vi "ReOrigin.vi"() -> ()   [LabVIEW 2018]
uses:
  <vilib>/Utility/miscctls.llb/LVPointTypeDef.ctl
  <vilib>/Utility/error.llb/DialogType.ctl
panel:
  in  "控件排布前面板.位置_前.位置":T1 caption="假设原点"
  in  "设定":bool
  out "Error Report":string
  out "Current State":string
  in  "Data Structure":T2
  in  "OK":bool
  in  "Exit Program":bool
  in  "Error":bool
  in  "Parameter":T3={"Q-HighLevel"="Q-HighLevel", "Q-Local"="Enginex", "Data"=variant}
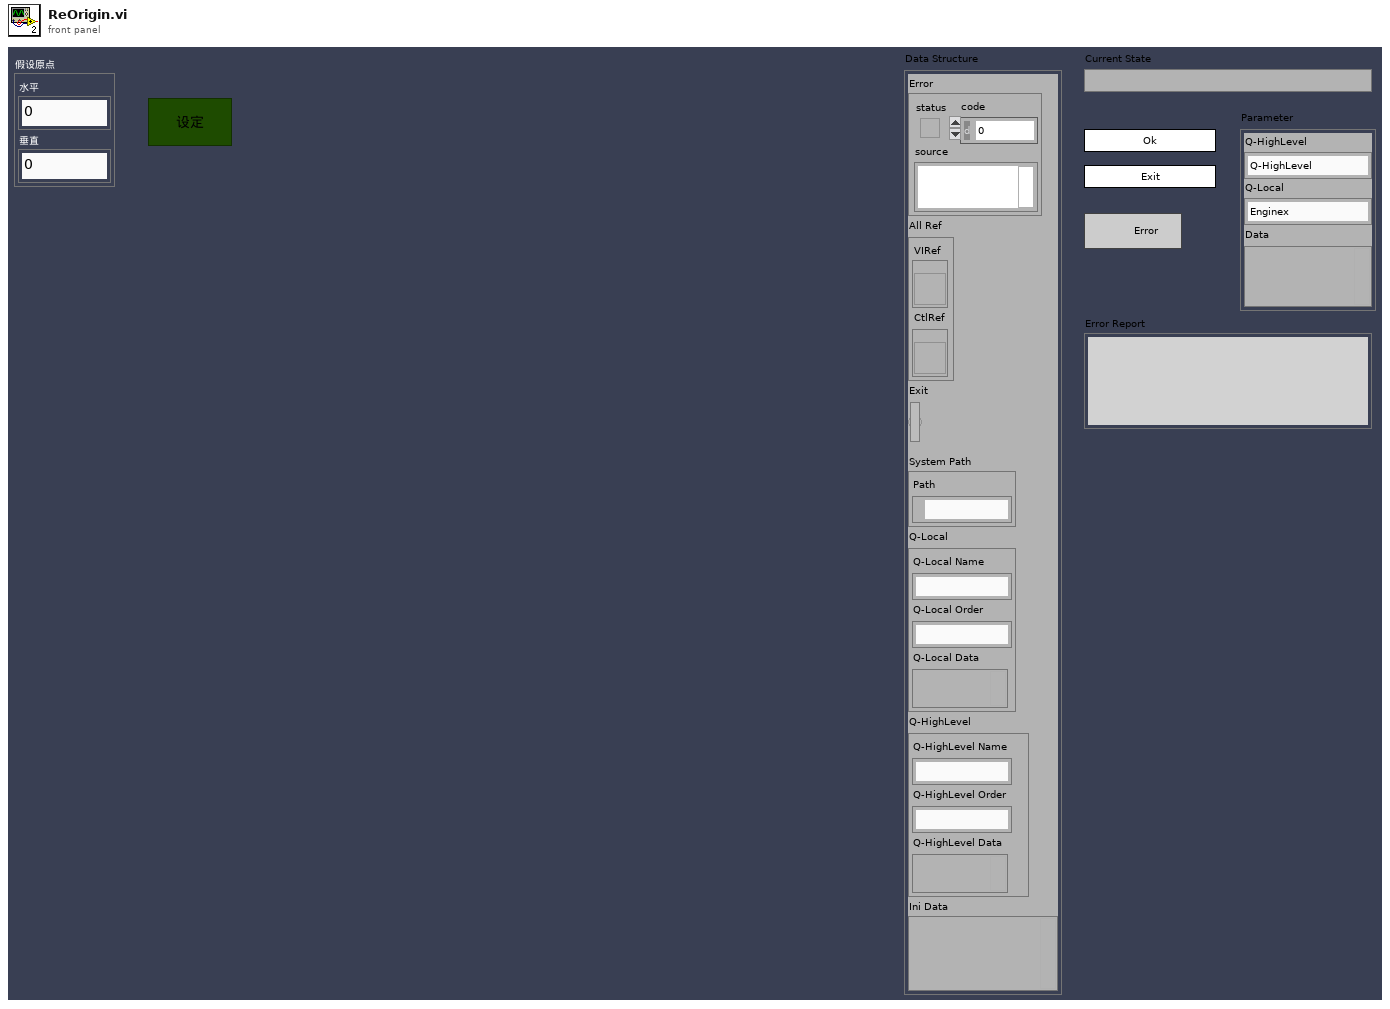
[diagram p1: front panel]
types:
  T1 = typedef "LVPointTypeDef.ctl" = cluster{"Horizontal":i16, "Vertical":i16}
  T2 = cluster{"Error":errorcluster, "All Ref":cluster{"VIRef":refnum<vi>, "CtlRef":refnum<vi>}, "Exit":bool, "System Path":cluster{"Path":path}, "Q-Local":cluster{"Q-Local Name":string, "Q-Local Order":string, "Q-Local Data":variant}, "Q-HighLevel":cluster{"Q-HighLevel Name":string, "Q-HighLevel Order":string, "Q-HighLevel Data":variant}, "Ini Data":variant}
  T3 = cluster{"Q-HighLevel":string, "Q-Local":string, "Data":variant}
  T4 = typedef "eventvkey.ctl" = enum16{"ASCII", "Enter", "Return", "Shift", "Ctrl", "Alt", "Cmd", "Opt", "Caps", "NumLock", "Clear", "Break", "Up", "Down", "Left", "Right", "Insert", "Delete", "Home", "End", "PageUp", "PageDown", "Escape", "Help", "Pause", "ScrollLock", "F1", "F2", "F3", "F4", "F5", "F6", "F7", "F8", "F9", "F10", "F11", "F12", "F13", "F14", "F15", "F16", "F17", "F18", "F19", "F20", "F21", "F22", "F23", "F24", "Play", "VolumeUp", "VolumeDown", "Mute", "Two Byte Char"}
  T5 = typedef "DialogType.ctl" = u16
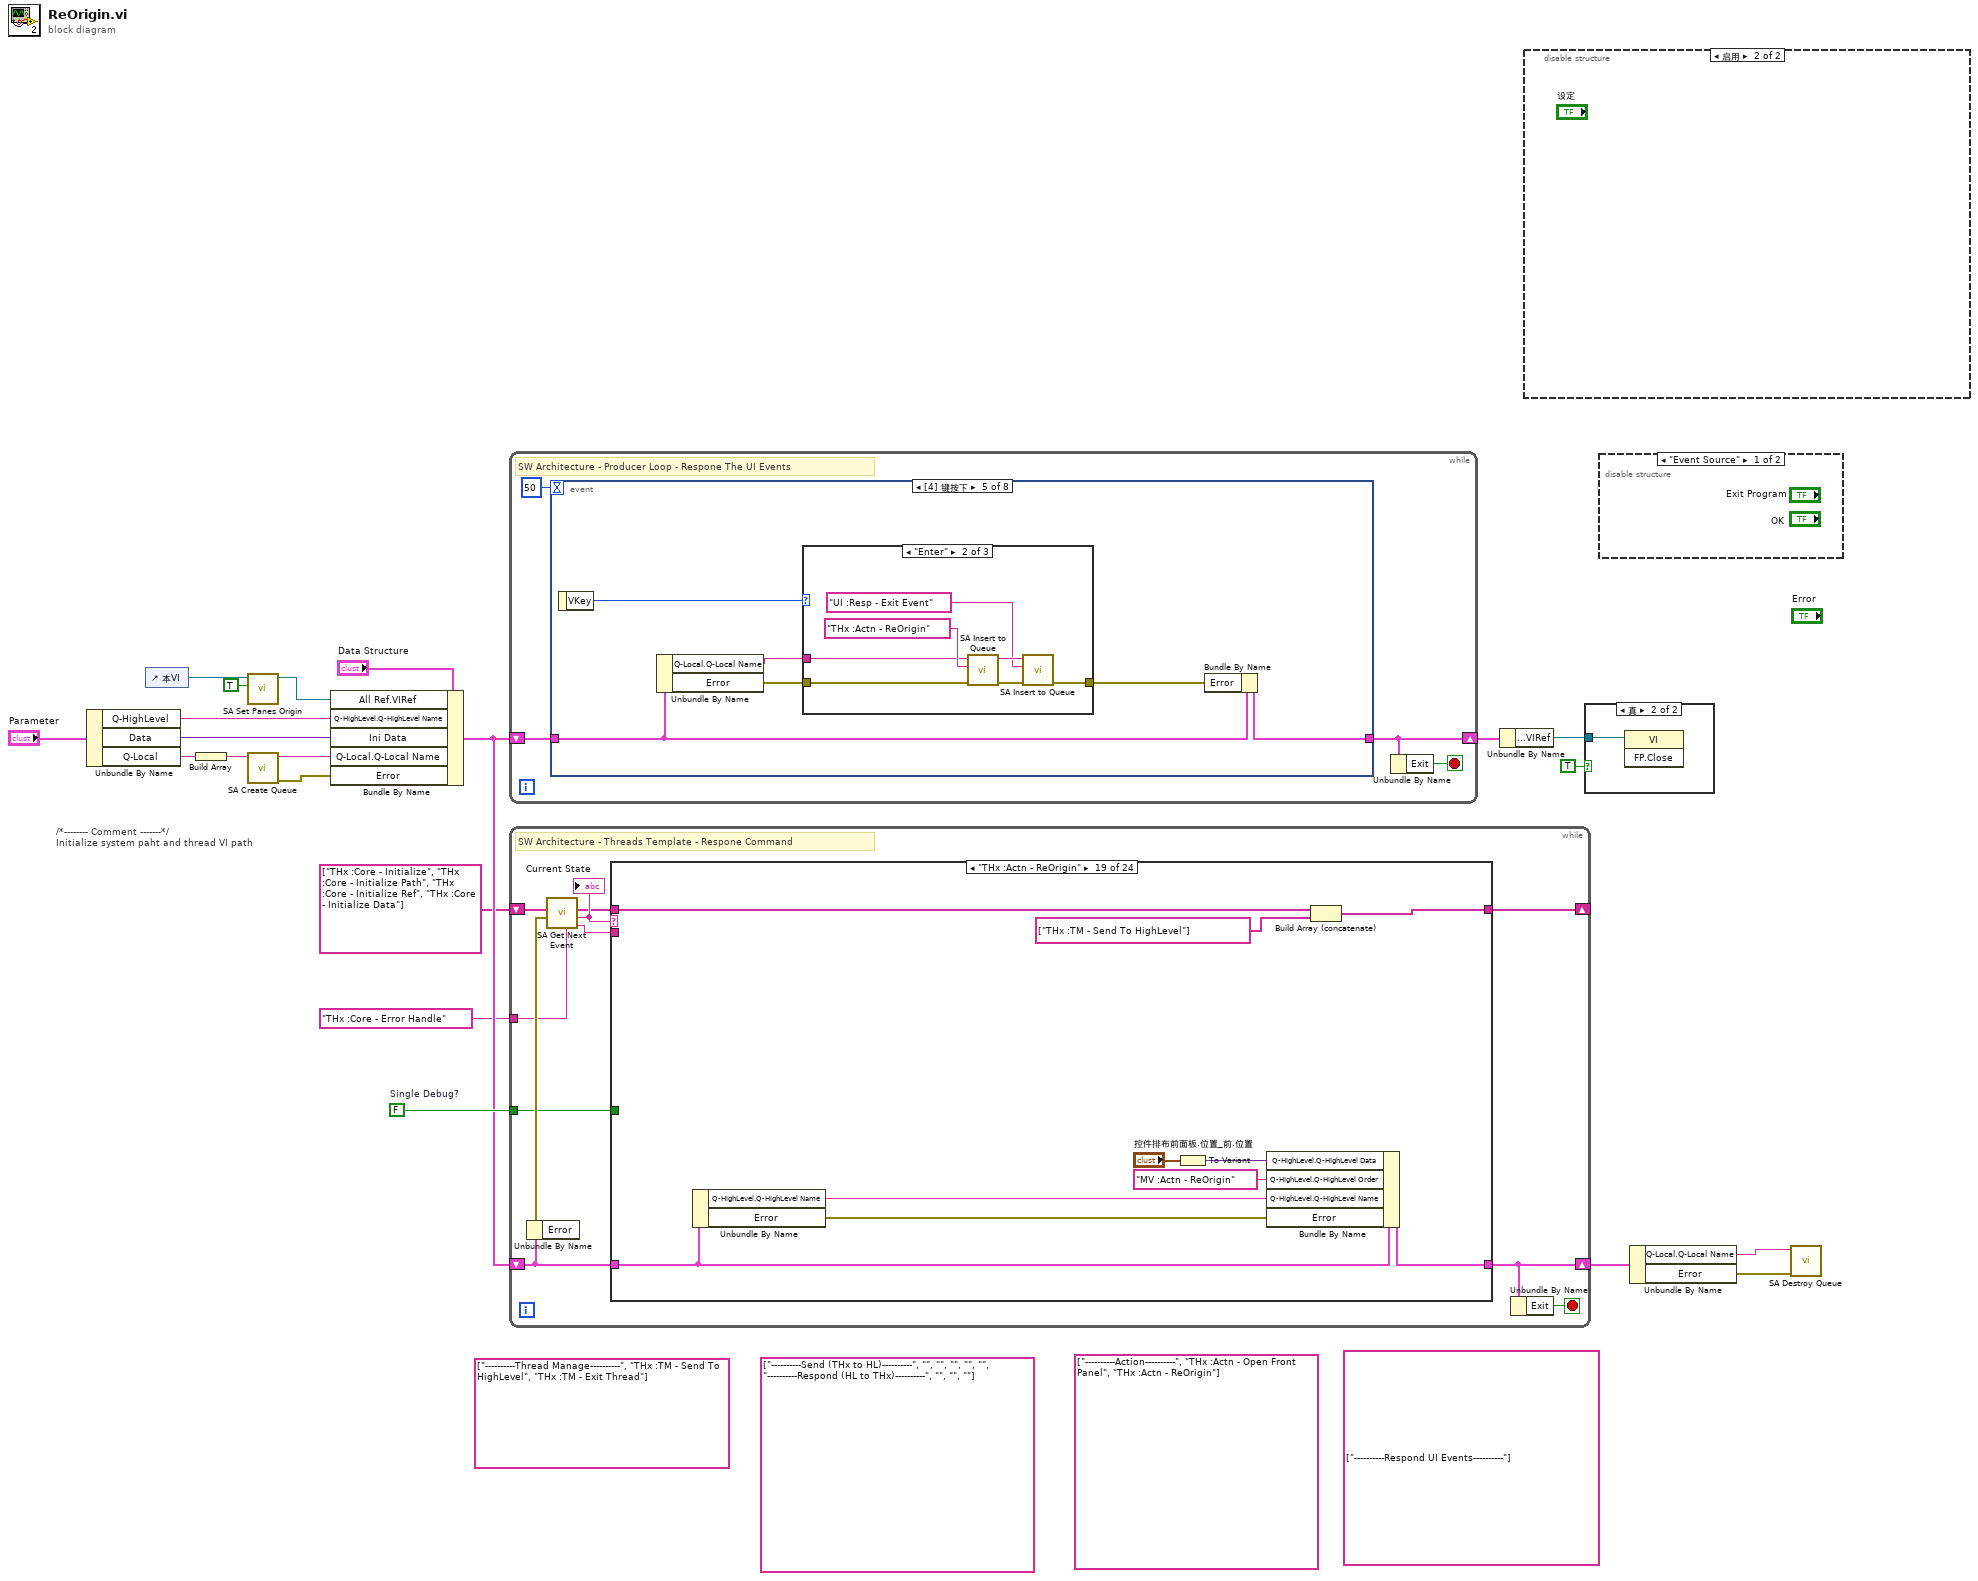
[diagram p0: block diagram]
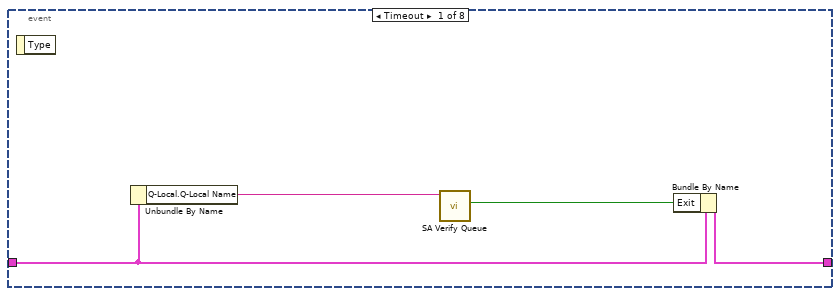
[diagram p5: hidden frame]
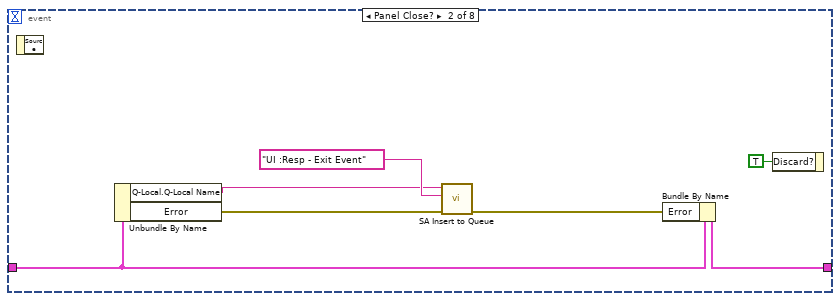
[diagram p6: hidden frame]
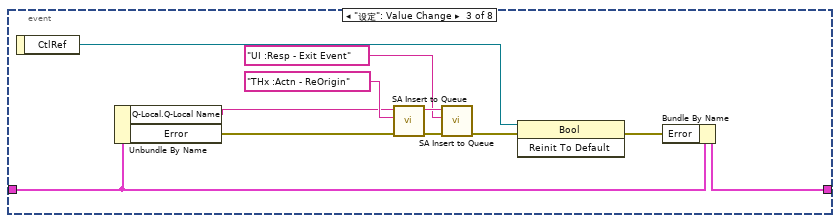
[diagram p7: hidden frame]
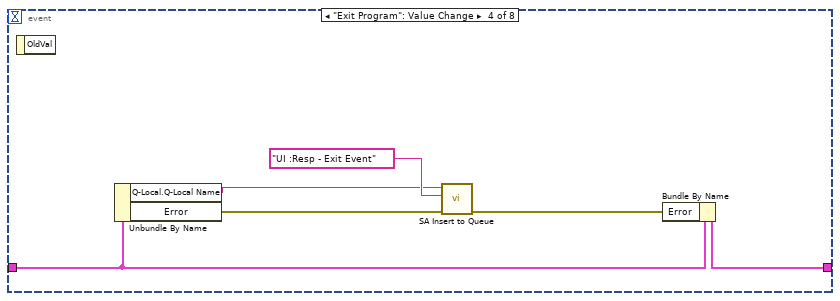
[diagram p8: hidden frame]
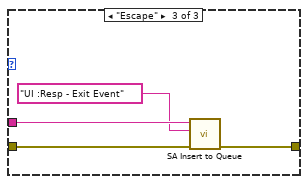
[diagram p10: hidden frame]
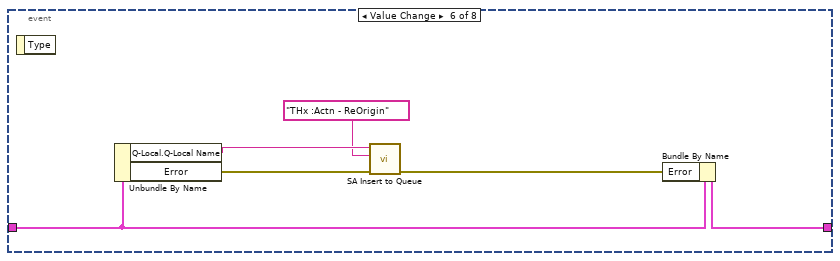
[diagram p11: hidden frame]
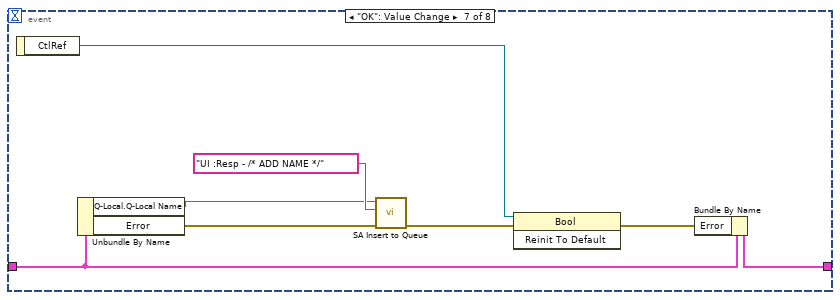
[diagram p12: hidden frame]
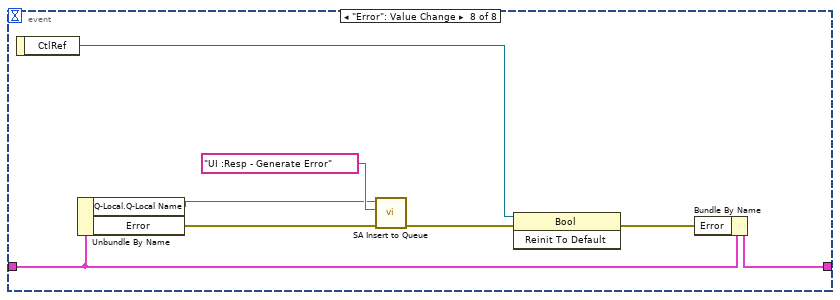
[diagram p13: hidden frame]
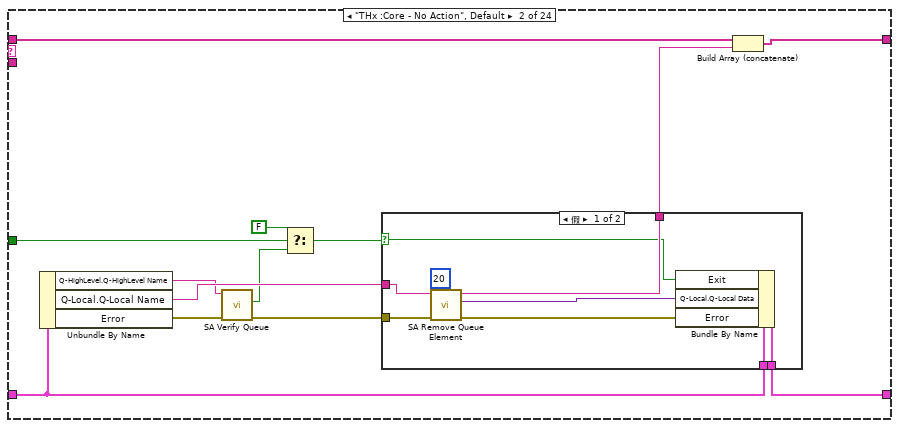
[diagram p15: hidden frame]
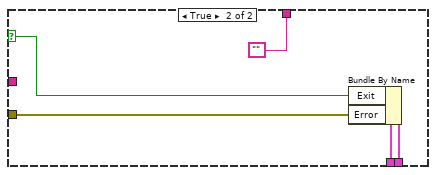
[diagram p16: hidden frame]
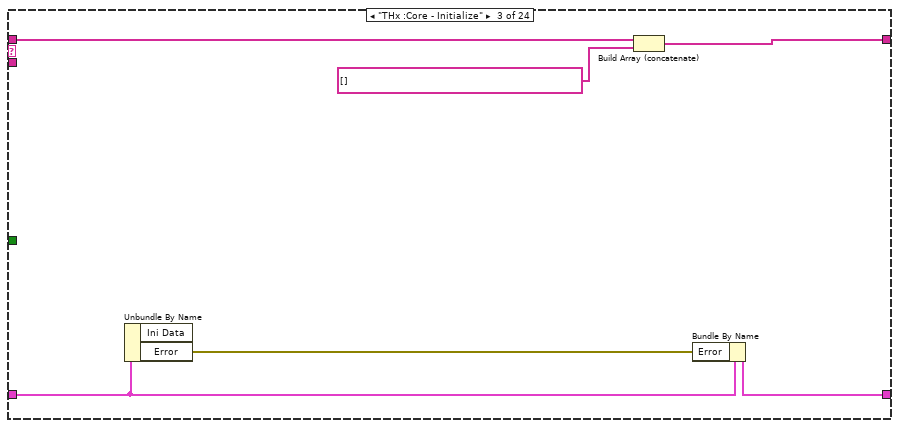
[diagram p17: hidden frame]
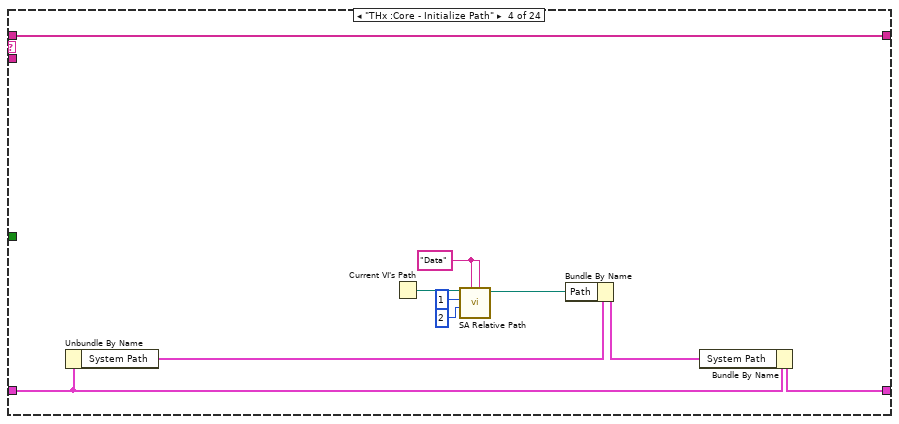
[diagram p18: hidden frame]
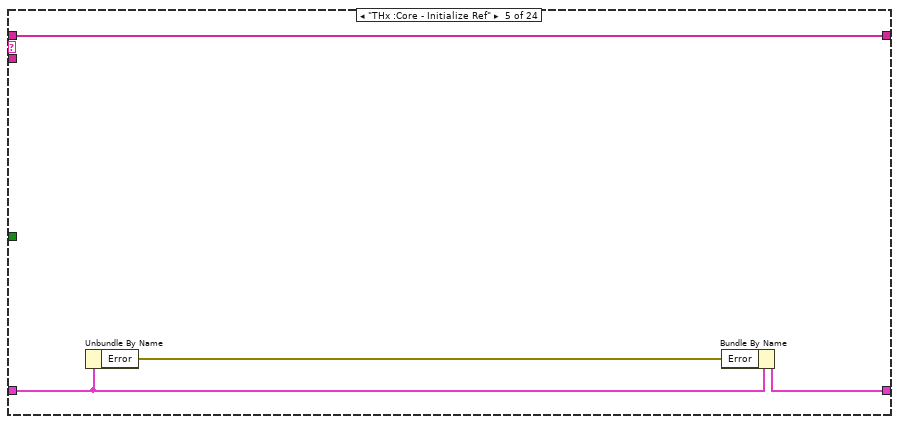
[diagram p19: hidden frame]
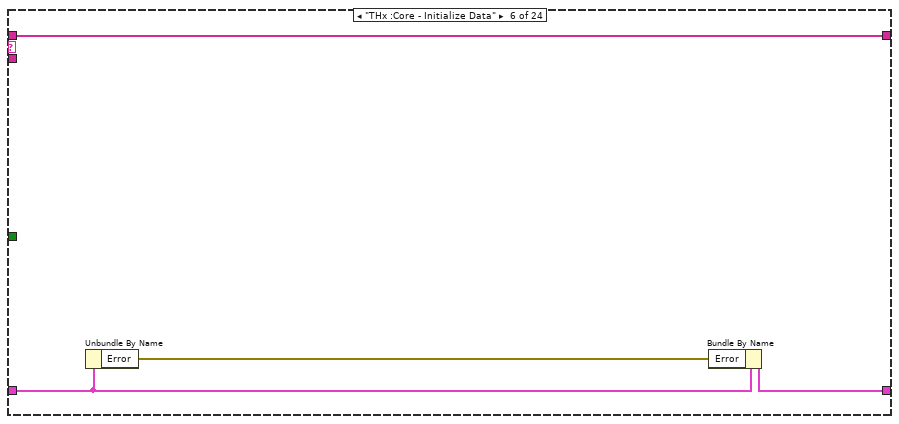
[diagram p20: hidden frame]
diagram:
  w16 = FALSE  # Single Debug?
  (unwired) string[] ["----------Action----------", "THx :Actn - Open Front Panel", "THx :Actn - ReOrigin"]
  (unwired) string[] ["----------Respond UI Events----------"]
  (unwired) string[] ["----------Send (THx to HL)----------", "", "", "", "", "", "----------Respond (HL to THx)----------", "", "", ""]
  (unwired) string[] ["----------Thread Manage----------", "THx :TM - Send To HighLevel", "THx :TM - Exit Thread"]
  # "/*-------- Comment -------*/\nInitialize system paht and thread VI path"
  n1 = Unbundle By Name("Parameter") -> ("Q-HighLevel"=w15:string, "Data"=w17:variant, "Q-Local"=w14:string)
  n2 = control-ref of="本VI"() -> (w18:refnum<vi>)
  n3 = Build Array(w14) -> (w12:string[])
  n4 = call <vilib>:"SA Set Panes Origin.vi"("Enable? (F)"=TRUE, "VI Ref in"=w18) -> ("VI Ref out"=w19:refnum<vi>)  [unwired: 9 in]
  n5 = call <vilib>:"SA Create Queue.vi"("Queue Name"=w12) -> ("error out"=w7:errorcluster)  [unwired: 10 in]
  n6 = Bundle By Name(cluster="Data Structure", "All Ref.VIRef"=w19, "Q-HighLevel.Q-HighLevel Name"=w15, "Ini Data"=w17, "Q-Local.Q-Local Name"=w14, "Error"=w7) -> (w8:T2)
  n7 = while {
    shift-right: [w22] -> w9
    shift-left: w8 -> [w23]
    stop <- w21 stop-if-true
    # "SW Architecture - Producer Loop - Respone The UI Events"
    n8 = event shown="[4] 键按下" {
      selector: _ -> [_ _ _ _ _ _ _ _]
      dyn-events: _ -> [_ _ _ _ _ _ _ _]
      timeout: 50 -> [_ _ _ _ _ _ _ _]
      tunnel: w23 -> [w26 w33 w43 w49 w56 w73 w77 w85]
      tunnel: [w28 w32 w42 w48 w55 w72 w76 w84] -> w22
      event Timeout {
        n9 = event-data() -> ()  [unwired: 1 in, 1 out]
        n10 = Unbundle By Name(w26) -> ("Q-Local.Q-Local Name"=w25:string)
        n11 = call <vilib>:"SA Verify Queue.vi"("Queue Name in"=w25) -> ("Not A Queue?"=w27:bool)  [unwired: 6 in, 3 out]
        n12 = Bundle By Name(cluster=w26, "Exit"=w27) -> (w28:T2)
      }
      event Panel Close? {
        n13 = event-data() -> ()  [unwired: 1 in, 1 out]
        n14 = Unbundle By Name(w33) -> ("Q-Local.Q-Local Name"=w30:string, "Error"=w34:errorcluster)
        n15 = call <vilib>:"SA Insert to Queue.vi"("error in"=w34, "Event"="UI :Resp - Exit Event", "Queue Name"=w30) -> ("error out"=w31:errorcluster)  [unwired: 8 in]
        n16 = Bundle By Name(cluster=w33, "Error"=w31) -> (w32:T2)
        n17 = event-data("Discard?"=TRUE ("放弃？")) -> ()  [unwired: 1 in, 1 out]
      }
      event "设定": Value Change {
        n18 = event-data() -> ("CtlRef"=w40:refnum<vi>)  [unwired: 1 in]
        n19 = Unbundle By Name(w43) -> ("Q-Local.Q-Local Name"=w37:string, "Error"=w44:errorcluster)
        n20 = call <vilib>:"SA Insert to Queue.vi"("error in"=w44, "Event"="THx :Actn - ReOrigin", "Queue Name"=w37) -> ("error out"=w39:errorcluster)  [unwired: 8 in]
        n21 = call <vilib>:"SA Insert to Queue.vi"("error in"=w39, "Event"="UI :Resp - Exit Event", "Queue Name"=w37) -> ("error out"=w38:errorcluster)  [unwired: 8 in]
        n22 = invoke class="Bool" method="Reinit To Default"(reference=w40, error in=w38) -> (error out=w41:errorcluster)  [unwired: 1 in, 2 out]
        n23 = Bundle By Name(cluster=w43, "Error"=w41) -> (w42:T2)
      }
      event "Exit Program": Value Change {
        n24 = event-data() -> ()  [unwired: 1 in, 1 out]
        n25 = Unbundle By Name(w49) -> ("Q-Local.Q-Local Name"=w46:string, "Error"=w50:errorcluster)
        n26 = call <vilib>:"SA Insert to Queue.vi"("error in"=w50, "Event"="UI :Resp - Exit Event", "Queue Name"=w46) -> ("error out"=w47:errorcluster)  [unwired: 8 in]
        n27 = Bundle By Name(cluster=w49, "Error"=w47) -> (w48:T2)
      }
      event Key Down {
        n28 = event-data() -> ("VKey"=w52:T4)  [unwired: 1 in]
        n29 = Unbundle By Name(w56) -> ("Q-Local.Q-Local Name"=w53:string, "Error"=w57:errorcluster)
        n30 = case shown="\"Enter\"" w52 {
          tunnel: w57 -> [w58 w64 w68]
          tunnel: [w58 w61 w67] -> w54
          tunnel: w53 -> [_ w60 w66]
          frame "ASCII", Default {
          }
          frame "Enter" {
            n31 = call <vilib>:"SA Insert to Queue.vi"("error in"=w64, "Event"="THx :Actn - ReOrigin", "Queue Name"=w60) -> ("error out"=w62:errorcluster)  [unwired: 8 in]
            n32 = call <vilib>:"SA Insert to Queue.vi"("error in"=w62, "Event"="UI :Resp - Exit Event", "Queue Name"=w60) -> ("error out"=w61:errorcluster)  [unwired: 8 in]
          }
          frame "Escape" {
            n33 = call <vilib>:"SA Insert to Queue.vi"("error in"=w68, "Event"="UI :Resp - Exit Event", "Queue Name"=w66) -> ("error out"=w67:errorcluster)  [unwired: 8 in]
          }
        }
        n34 = Bundle By Name(cluster=w56, "Error"=w54) -> (w55:T2)
      }
      event Value Change {
        n35 = event-data() -> ()  [unwired: 1 in, 1 out]
        n36 = Unbundle By Name(w73) -> ("Q-Local.Q-Local Name"=w71:string, "Error"=w74:errorcluster)
        n37 = call <vilib>:"SA Insert to Queue.vi"("error in"=w74, "Event"="THx :Actn - ReOrigin", "Queue Name"=w71) -> ("error out"=w69:errorcluster)  [unwired: 8 in]
        n38 = Bundle By Name(cluster=w73, "Error"=w69) -> (w72:T2)
      }
      event "OK": Value Change {
        n39 = event-data() -> ("CtlRef"=w82:refnum<vi>)  [unwired: 1 in]
        n40 = Unbundle By Name(w77) -> ("Q-Local.Q-Local Name"=w75:string, "Error"=w80:errorcluster)
        n41 = call <vilib>:"SA Insert to Queue.vi"("error in"=w80, "Event"="UI :Resp - /* ADD NAME */", "Queue Name"=w75) -> ("error out"=w79:errorcluster)  [unwired: 8 in]
        n42 = invoke class="Bool" method="Reinit To Default"(reference=w82, error in=w79) -> (error out=w78:errorcluster)  [unwired: 1 in, 2 out]
        n43 = Bundle By Name(cluster=w77, "Error"=w78) -> (w76:T2)
      }
      event "Error": Value Change {
        n44 = event-data() -> ("CtlRef"=w90:refnum<vi>)  [unwired: 1 in]
        n45 = Unbundle By Name(w85) -> ("Q-Local.Q-Local Name"=w83:string, "Error"=w88:errorcluster)
        n46 = call <vilib>:"SA Insert to Queue.vi"("error in"=w88, "Event"="UI :Resp - Generate Error", "Queue Name"=w83) -> ("error out"=w87:errorcluster)  [unwired: 8 in]
        n47 = invoke class="Bool" method="Reinit To Default"(reference=w90, error in=w87) -> (error out=w86:errorcluster)  [unwired: 1 in, 2 out]
        n48 = Bundle By Name(cluster=w85, "Error"=w86) -> (w84:T2)
      }
    }
    n49 = Unbundle By Name(w22) -> ("Exit"=w21:bool)
  }
  n50 = while {
    shift-right: [w95] -> w6
    shift-left: w8 -> [w97]
    shift-right: [w98] -> _
    shift-left: string[] ["THx :Core - Initialize", "THx :Core - Initialize Path", "THx :Core - Initialize Ref", "THx :Core - Initialize Data"] -> [w101]
    tunnel: "THx :Core - Error Handle" ("Error Handle") -> [w93]
    tunnel: w16 -> [w91]
    stop <- w94 stop-if-true
    # "SW Architecture - Threads Template - Respone Command"
    n51 = Unbundle By Name(w97) -> ("Error"=w96:errorcluster)
    n52 = call <vilib>:"SA Get Next Event.vi"("Error Handle"=w93, "error in"=w96, "event queue in"=w101) -> ("prev event"=w92:string, "next event"=w100:string, "event queue out"=w99:string[])  [unwired: 6 in]
    "Current State" <- w100
    n53 = case shown="\"THx :Actn - ReOrigin\"" w100 {
      tunnel: w97 -> [w102 w116 w134 w144 w148 w152 w167 w170 w174 w181 w195 w201 w206 w208 w213 w219 w221 w226 w236 w242 w244 w249 w255 w260]
      tunnel: w99 -> [w103 w114 w136 w146 w150 w154 _ w173 w175 w184 w200 w202 w207 w209 w214 w217 w222 w227 w237 w243 w245 w247 w253 w258]
      tunnel: [w103 w113 w135 w146 w150 w154 string[] ["THx :TM - Send To HighLevel"] w173 w175 w184 w199 w202 w203 w209 w210 w216 w222 w223 w233 w243 w245 w246 w252 w257] -> w98
      tunnel: [w102 w115 w133 w145 w149 w153 w168 w171 w174 w180 w197 w201 w204 w208 w211 w218 w221 w225 w235 w241 w244 w248 w254 w259] -> w95
      tunnel: w92 -> [_ _ _ _ _ _ w163 _ _ _ _ _ _ _ _ _ _ _ _ _ _ _ _ _]
      tunnel: w91 -> [_ w108 _ _ _ _ _ _ _ _ _ _ _ _ _ _ _ _ _ _ _ _ _ _]
      frame "----------Core Status----------" {
      }
      frame "THx :Core - No Action", Default {
        n54 = Unbundle By Name(w116) -> ("Q-HighLevel.Q-HighLevel Name"=w105:string, "Q-Local.Q-Local Name"=w111:string, "Error"=w110:errorcluster)
        n55 = call <vilib>:"SA Verify Queue.vi"("error in"=w110, "Queue Name in"=w105) -> ("error out"=w109:errorcluster, "Not A Queue?"=w104:bool)  [unwired: 5 in, 2 out]
        n56 = Select(t=FALSE, s=w108, f=w104) -> (s? t:f=w106:bool)
        n57 = case shown="假" w106 {
          selector: w106 -> [w117 w128]
          tunnel: w116 -> [w123 w129]
          tunnel: [w122 w126] -> w115
          tunnel: [w121 "" ("Event")] -> w112
          tunnel: w111 -> [w119 _]
          tunnel: w109 -> [w118 w127]
          frame False {
            n58 = call <vilib>:"SA Remove Queue Element.vi"("Time out (10)"=20 ("Time out(-1)_queue out"), "error in"=w118, "Queue Name"=w119) -> ("error out"=w125:errorcluster, "Data"=w124:variant, "Event"=w121:string)  [unwired: 5 in, 1 out]
            n59 = Bundle By Name(cluster=w123, "Exit"=w117, "Q-Local.Q-Local Data"=w124, "Error"=w125) -> (w122:T2)
          }
          frame True {
            n60 = Bundle By Name(cluster=w129, "Exit"=w128, "Error"=w127) -> (w126:T2)
          }
        }
        n61 = Build Array (concatenate)(w114, w112) -> (w113:string[])
      }
      frame "THx :Core - Initialize" {
        n62 = Unbundle By Name(w134) -> ("Error"=w132:errorcluster)  [unwired: 1 out]
        n63 = Build Array (concatenate)(w136, string[] [] ("数组")) -> (w135:string[])
        n64 = Bundle By Name(cluster=w134, "Error"=w132) -> (w133:T2)
      }
      frame "THx :Core - Initialize Path" {
        w139 = "Data" ("Data Folder Path")
        n65 = Unbundle By Name(w144) -> ("System Path"=w138:cluster{"Path":path})
        n66 = Current VI's Path() -> (path=w140:path)
        n67 = call <vilib>:"SA Relative Path.vi"("Development Relative Path"=w139, "Run Time Relative path"=w139, "Run-Time File Depth"=2, "Development File Depth"=1, "Root Path"=w140) -> ("Relative Path"=w143:path)  [unwired: 5 in, 1 out]
        n68 = Bundle By Name(cluster=w138, "Path"=w143) -> (w137:cluster{"Path":path})
        n69 = Bundle By Name(cluster=w144, "System Path"=w137) -> (w145:T2)
      }
      frame "THx :Core - Initialize Ref" {
        n70 = Unbundle By Name(w148) -> ("Error"=w147:errorcluster)
        n71 = Bundle By Name(cluster=w148, "Error"=w147) -> (w149:T2)
      }
      frame "THx :Core - Initialize Data" {
        n72 = Unbundle By Name(w152) -> ("Error"=w151:errorcluster)
        n73 = Bundle By Name(cluster=w152, "Error"=w151) -> (w153:T2)
      }
      frame "THx :Core - Error Handle" {
        w164 = T5 2 items=["no dialog", "OK message", "continue or stop message", "OK message + warnings", "continue/stop + warnings"] ("type of dialog (OK msg:1)")
        n74 = Unbundle By Name(w167) -> ("Error.source"=w161:string, "Error"=w165:errorcluster)
        n75 = call <vilib>:"Simple Error Handler.vi"("type of dialog (OK msg:1)"=w164, "error in (no error)"=w165) -> ("error out"=w157:errorcluster, "message"=w160:string)  [unwired: 3 in, 3 out]
        n76 = Concatenate Strings(w163, " -> " ("字符串"), w161, w160) -> (→"Error Report":string)
        n77 = To Variant(anything=w157) -> (Variant=w156:variant)
        n78 = call <vilib>:"Clear Errors.vi"("error in (no error)"=w157) -> ("error out"=w166:errorcluster)  [unwired: 5 in, 1 out]
        n79 = Bundle By Name(cluster=w167, "Q-HighLevel.Q-HighLevel Order"="THx :TM - Return Error" ("Q-Local.Q-Local Order"), "Error"=w166, "Q-HighLevel.Q-HighLevel Data"=w156) -> (w168:T2)
      }
      frame "THx :Core - Exit Thread" {
        n80 = Unbundle By Name(w170) -> ("Error"=w172:errorcluster)
        n81 = Bundle By Name(cluster=w170, "Exit"=TRUE, "Error"=w172) -> (w171:T2)
      }
      frame "----------Thread Manage----------" {
      }
      frame "THx :TM - Send To HighLevel" {
        n82 = Unbundle By Name(w181) -> ("Q-HighLevel.Q-HighLevel Name"=w183:string, "Q-HighLevel.Q-HighLevel Order"=w178:string, "Q-HighLevel.Q-HighLevel Data"=w177:variant, "Error"=w182:errorcluster)
        n83 = call <vilib>:"SA Verify Queue.vi"("Queue Name in"=w183) -> ("Not A Queue?"=w179:bool)  [unwired: 6 in, 3 out]
        n84 = case shown="假" w179 {
          tunnel: w182 -> [w190 w191]
          tunnel: w183 -> [w189 _]
          tunnel: w178 -> [w187 _]
          tunnel: w177 -> [w188 _]
          tunnel: [w186 w191] -> w176
          frame False {
            n85 = call <vilib>:"SA Insert to Queue.vi"("Time out (10)"=50 ("Time out(-1)_queue in"), "error in"=w190, "Data"=w188, "Event"=w187, "Queue Name"=w189) -> ("error out"=w186:errorcluster)  [unwired: 6 in]
          }
          frame True {
          }
        }
        n86 = Bundle By Name(cluster=w181, "Error"=w176) -> (w180:T2)
      }
      frame "THx :TM - Exit Thread" {
        n87 = Unbundle By Name(w195) -> ("Q-Local.Q-Local Name"=w194:string, "Error"=w192:errorcluster)
        n88 = To Variant(anything=w194) -> (Variant=w193:variant)
        n89 = Bundle By Name(cluster=w195, "Q-HighLevel.Q-HighLevel Order"="THx :TM - Delete Dynamic Thread", "Q-HighLevel.Q-HighLevel Data"=w193, "Error"=w192) -> (w197:T2)
        n90 = Build Array (concatenate)(w200, string[] ["THx :TM - Send To HighLevel", "THx :Core - Exit Thread"] ("数组")) -> (w199:string[])
      }
      frame "----------Send (THx to HL)----------" {
      }
      frame "THx :HL - /* ADD NAME */" {
        n91 = Unbundle By Name(w206) -> ("Error"=w205:errorcluster)
        n92 = Build Array (concatenate)(w207) -> (w203:string[])
        n93 = Bundle By Name(cluster=w206, "Error"=w205) -> (w204:T2)
      }
      frame "----------Respond (HL to THx)----------" {
      }
      frame "HL :THx - /* ADD NAME */" {
        n94 = Unbundle By Name(w213) -> ("Error"=w212:errorcluster)
        n95 = Build Array (concatenate)(w214) -> (w210:string[])
        n96 = Bundle By Name(cluster=w213, "Error"=w212) -> (w211:T2)
      }
      frame "TM :THx - Quit Dynamic Thread" {
        n97 = Unbundle By Name(w219) -> ("Error"=w220:errorcluster)
        n98 = Bundle By Name(cluster=w219, "Error"=w220) -> (w218:T2)
        n99 = Build Array (concatenate)(w217, string[] ["THx :TM - Exit Thread"] ("数组")) -> (w216:string[])
      }
      frame "----------Actions----------" {
      }
      frame "THx :Actn - /* ADD NAME */" {
        n100 = Unbundle By Name(w226) -> ("Error"=w224:errorcluster)
        n101 = Build Array (concatenate)(w227) -> (w223:string[])
        n102 = Bundle By Name(cluster=w226, "Error"=w224) -> (w225:T2)
      }
      frame "THx :Actn - ReOrigin" {
        n103 = Unbundle By Name(w236) -> ("Q-HighLevel.Q-HighLevel Name"=w232:string, "Error"=w234:errorcluster)
        n104 = To Variant(anything="控件排布前面板.位置_前.位置") -> (Variant=w230:variant)
        n105 = Bundle By Name(cluster=w236, "Q-HighLevel.Q-HighLevel Data"=w230, "Q-HighLevel.Q-HighLevel Order"="MV :Actn - ReOrigin", "Q-HighLevel.Q-HighLevel Name"=w232, "Error"=w234) -> (w235:T2)
        n106 = Build Array (concatenate)(w237, string[] ["THx :TM - Send To HighLevel"] ("数组")) -> (w233:string[])
      }
      frame "THx :Actn - Open Front Panel" {
        n107 = Unbundle By Name(w242) -> ("All Ref.VIRef"=w238:refnum<vi>, "Error"=w240:errorcluster)
        n108 = invoke class="VI" method="FP.Open"(reference=w238, error in=w240) -> (error out=w239:errorcluster)  [unwired: 3 in, 4 out]
        n109 = Bundle By Name(cluster=w242, "Error"=w239) -> (w241:T2)
      }
      frame "----------Respond Events----------" {
      }
      frame "UI :Resp - /* ADD NAME */" {
        n110 = Unbundle By Name(w249) -> ("Error"=w250:errorcluster)
        n111 = Build Array (concatenate)(w247) -> (w246:string[])
        n112 = Bundle By Name(cluster=w249, "Error"=w250) -> (w248:T2)
      }
      frame "UI :Resp - Generate Error" {
        n113 = Unbundle By Name(w255) -> ()  [unwired: 1 out]
        n114 = Build Array (concatenate)(w253) -> (w252:string[])
        n115 = Bundle By Name(cluster=w255, "Error"=errorcluster {"status"=TRUE, "code"=-1, "source"="Error Test"}) -> (w254:T2)
      }
      frame "UI :Resp - Exit Event" {
        n116 = Unbundle By Name(w260) -> ("Error"=w261:errorcluster)
        n117 = Build Array (concatenate)(w258, string[] ["THx :TM - Exit Thread"] ("数组")) -> (w257:string[])
        n118 = Bundle By Name(cluster=w260, "Error"=w261) -> (w259:T2)
      }
    }
    n119 = Unbundle By Name(w95) -> ("Exit"=w94:bool)
  }
  n120 = Unbundle By Name(w9) -> ("All Ref.VIRef"=w10:refnum<vi>)
  n121 = disable-structure shown="启用" {
    frame Disabled {
    }
    frame Enabled {
    }
  }
  n122 = case shown="真" TRUE {
    tunnel: w10 -> [_ w262]
    frame False {
    }
    frame True {
      n123 = invoke class="VI" method="FP.Close"(reference=w262) -> ()  [unwired: 2 in, 3 out]
    }
  }
  n124 = disable-structure shown="\"Event Source\"" {
    frame condition #0 (active) {
    }
    frame condition #1 {
    }
  }
  n125 = Unbundle By Name(w6) -> ("Q-Local.Q-Local Name"=w4:string, "Error"=w5:errorcluster)
  n126 = call <vilib>:"SA Destroy Queue.vi"("error in"=w5, "Queue Name"=w4) -> ()  [unwired: 9 in, 1 out]
